vi "Get Sink Info.vi"(4 "Sink Name":string, 8 "error in (no error)":errorcluster, 11 "Application Log in":refnum<class "Application Log.lvclass">) -> (0 "error out":errorcluster, 3 "Application Log out":refnum<class "Application Log.lvclass">)   [LabVIEW 2016, in "Stream Log.lvlib" / "Application Log.lvclass"]
doc: "--\nCopyright © 2017 Composed SystemsI All rights reserved.\n\nAuthor: Jon McBee <jon.mcbee@composed.io>\n\nThis library is provided \"AS IS\" ,WITHOUT WARRANTIES OR\nCONDITIONS OF ANY KIND, either express or implied.\n\nComposed Systems -- composed.io\n\nStream 0.0.1.1\nJon McBee - Composed Systems\nCopyright (c) 2017, Composed Systems"
uses:
  <userlib>/Composed Systems/Stream/Log/Application Log/Application Log.lvclass
  <userlib>/Composed Systems/Stream/Log/Application Log/Application Log.lvclass/Application Log.ctl
  <userlib>/Composed Systems/Stream/Log/Sink Look Up Table/Sink Look Up Table.lvclass
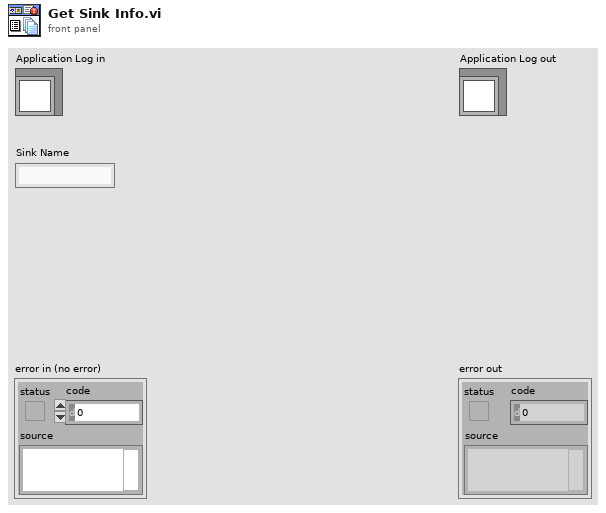
[diagram p1: front panel]
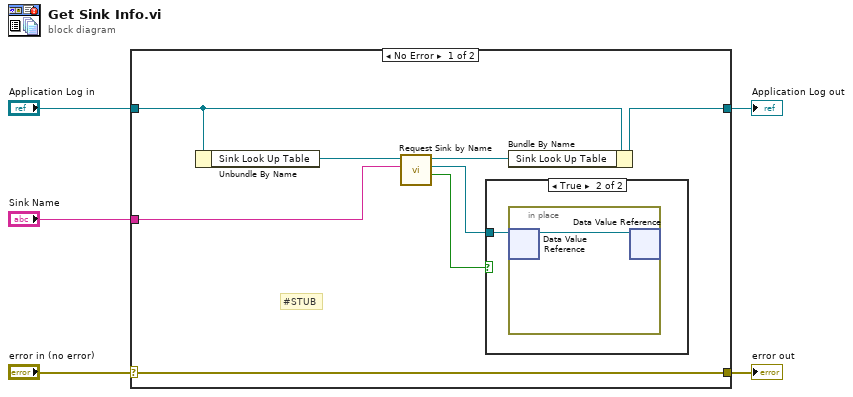
[diagram p0: block diagram]
diagram:
  n1 = case shown="No Error" "error in (no error)" {
    selector: "error in (no error)" -> [w13 w17]
    tunnel: [w13 w17] -> w4
    tunnel: [w8 w16] -> w2
    tunnel: "Application Log in" -> [w9 w16]
    tunnel: "Sink Name" -> [w11 _]
    frame No Error {
      # "#STUB"
      n2 = Unbundle By Name(w9) -> ("Sink Look Up Table"=w12:refnum<class "Sink Look Up Table.lvclass">)
      n3 = call <userlib>:"Request Sink by Name.vi"("Sink Name"=w11, "Sink Look Up Table in"=w12) -> ("Found?"=w6:bool, "Log Sink"=w7:refnum<data-value>, "Sink Look Up Table out"=w10:refnum<class "Sink Look Up Table.lvclass">)  [unwired: 6 in, 1 out]
      n4 = case shown="True" w6 {
        tunnel: w7 -> [_ w14]
        frame False {
        }
        frame True {
          n5 = in-place {
            n6 = in-place-dvr #1(w14) -> (w15:refnum<class "Log Sink.lvclass">)  [unwired: 1 out]
            n7 = in-place-dvr #1(w15) -> ()  [unwired: 2 out]
          }
        }
      }
      n8 = Bundle By Name(cluster=w9, "Sink Look Up Table"=w10) -> (w8:refnum<class "Application Log.lvclass">)
    }
    frame Error {
    }
  }
  "error out" <- w4
  "Application Log out" <- w2
